vi "Reset Block (0-3).vi"() -> ()   [LabVIEW 2017]
panel:
  out "x-y*floor(x/y)":dbl
  in  "y":dbl
  in  "x":dbl
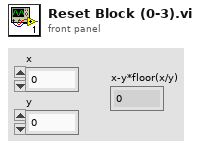
[diagram p1: front panel]
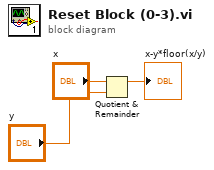
[diagram p0: block diagram]
diagram:
  n1 = Quotient & Remainder(x="x", y="y") -> (x-y*floor(x/y)=→"x-y*floor(x/y)":dbl)  [unwired: 1 out]
